vi "Configure Syringe Motion.vi"(8 "error in (no error)":errorcluster, 9 "Motion":T1={"Top Speed (5000 sps) "=5000, "Start Speed (750 sps)"=750, "Stop Speed (750 sps)"=750, "Acceleration (17500 steps/sec^2)"=17500, "Deceleration (17500 steps/sec^2)"=17500, "Backlash Steps (100 steps)"=100} {"Backlash Steps (100 steps)" max=1000 step=1; "Deceleration (17500 steps/sec^2)" min=2500 max=50000 step=2500; "Acceleration (17500 steps/sec^2)" min=2500 max=50000 step=2500; "Stop Speed (750 sps)" min=40 max=10000 step=1; "Start Speed (750 sps)" min=40 max=1000 step=1; "Top Speed (5000 sps)" min=40 max=10000 step=1}, 10 "Address (1)":u16=1 max=15 step=1, 11 "VISA resource name":refnum<visa-resource-name>) -> (0 "error out":errorcluster, 3 "VISA resource name out":refnum<visa-resource-name>)   [LabVIEW 2021, in "Copy of Kloehn V6 Series.lvlib"]
doc: "Configures the movement properties of the syringe for the instrument. Whenever the syringe moves, it will start at the top speed and accelerate until it reaches the top speed. When the syringe is close to completing the task, it will decelerate until it reaches its stop speed and then stops. Backlash steps is compensation for doing two different tasks that require opposite motion. Therefore, backlash is necessary when doing an dispense following an aspirate."
uses:
  Copy of Kloehn V6 Series.lvlib
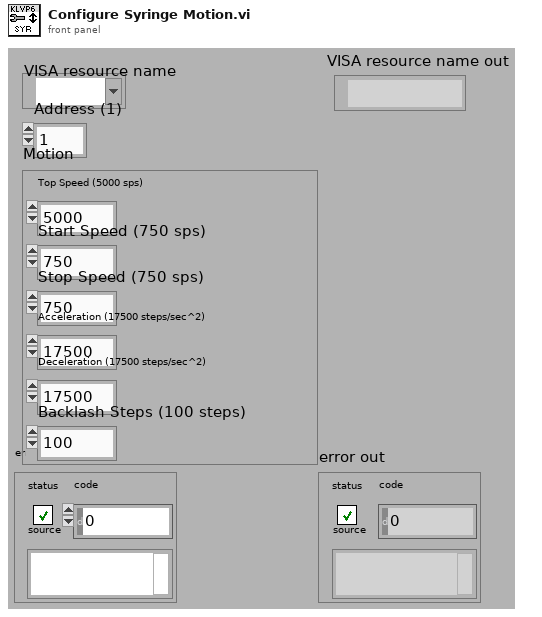
[diagram p1: front panel]
types:
  T1 = cluster{"Top Speed (5000 sps) ":u16, "Start Speed (750 sps)":u16, "Stop Speed (750 sps)":u16, "Acceleration (17500 steps/sec^2)":u16, "Deceleration (17500 steps/sec^2)":u16, "Backlash Steps (100 steps)":u16}
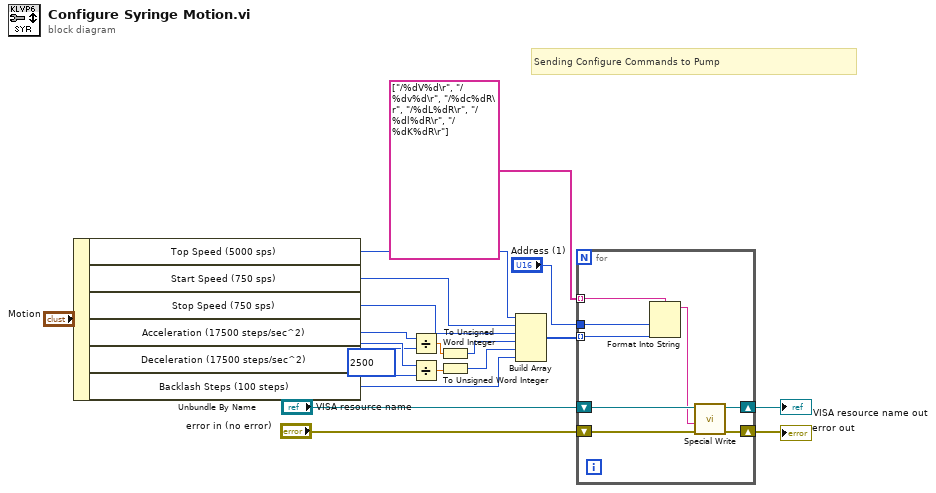
[diagram p0: block diagram]
diagram:
  w4 = u16 2500 ("y")
  # "Sending Configure Commands to Pump"
  n1 = Unbundle By Name("Motion") -> ("Top Speed (5000 sps)"=w10:u16, "Start Speed (750 sps)"=w9:u16, "Stop Speed (750 sps)"=w8:u16, "Acceleration (17500 steps/sec^2)"=w7:u16, "Deceleration (17500 steps/sec^2)"=w5:u16, "Backlash Steps (100 steps)"=w1:u16)
  n2 = Divide(x=w7, y=w4) -> (x/y=w15:dbl)
  n3 = Divide(x=w5, y=w4) -> (x/y=w14:dbl)
  n4 = To Unsigned Word Integer(number=w15) -> (unsigned 16bit integer=w3:u16)
  n5 = To Unsigned Word Integer(number=w14) -> (unsigned 16bit integer=w2:u16)
  n6 = Build Array(w10, w9, w8, w3, w2, w1) -> (w19:u16[])
  n7 = for {
    tunnel: w19 -> [w24] mode=indexing
    tunnel: string[] ["/%dV%d\r", "/%dv%d\r", "/%dc%dR\r", "/%dL%dR\r", "/%dl%dR\r", "/%dK%dR\r"] -> [w27] mode=indexing
    shift-right: [w20] -> w13
    shift-left: "error in (no error)" -> [w25]
    shift-right: [w21] -> w6
    shift-left: "VISA resource name" -> [w26]
    tunnel: "Address (1)" -> [w22]
    n8 = Format Into String(format string=w27, w22, w24) -> (resulting string=w23:string)  [unwired: 2 in, 1 out]
    n9 = call "Special Write.vi"("error in (no error)"=w25, "Send String"=w23, "VISA resource name"=w26) -> ("error out"=w20:errorcluster, "VISA resource name out"=w21:refnum<visa-resource-name>)  [unwired: 4 in, 3 out]
  }
  "error out" <- w13
  "VISA resource name out" <- w6
